vi "Digital_write_signal.vi"() -> ()   [LabVIEW 2020]
uses:
  <vilib>/DAQmx/write.llb/DAQmx Write (Digital 1D Bool NChan 1Samp 1Line).vi
  <vilib>/DAQmx/create/channels.llb/DAQmx Create Channel (DO-Digital Output).vi
  <vilib>/DAQmx/miscellaneous.llb/DAQmx Fill In Error Info.vi
panel:
  in  "Text Ring":u16(ring) items=["All Off", "488", "560", "595", "640"]
  in  "Stop":bool
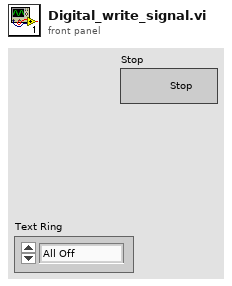
[diagram p1: front panel]
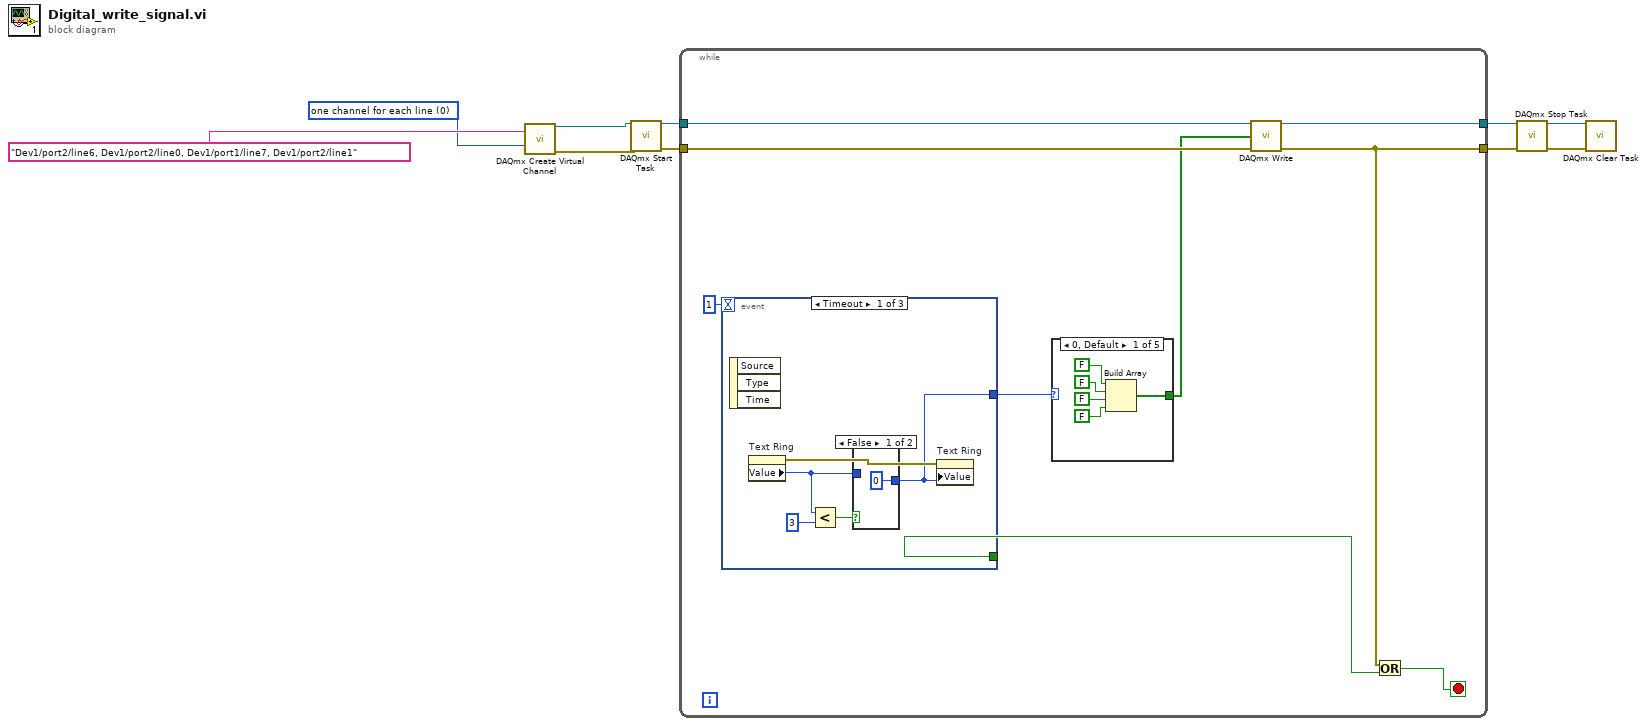
[diagram p0: block diagram]
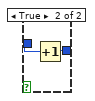
[diagram p2: hidden frame]
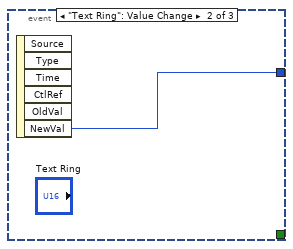
[diagram p3: hidden frame]
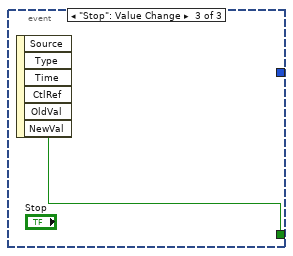
[diagram p4: hidden frame]
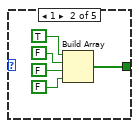
[diagram p5: hidden frame]
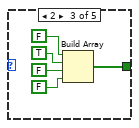
[diagram p6: hidden frame]
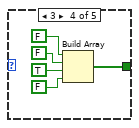
[diagram p7: hidden frame]
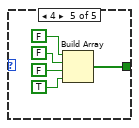
[diagram p8: hidden frame]
diagram:
  w1 = 0 items=["one channel for each line", "one channel for all lines"] ("line grouping")
  n1 = call-poly <vilib>:"DAQmx Create Virtual Channel.vi"("lines"=tag "Dev1/port2/line6, Dev1/port2/line0, Dev1/port1/line7, Dev1/port2/line1", "line grouping"=w1) -> ("task out"=w8:refnum<k21>, "error out"=w7:errorcluster)  [unwired: 12 in]
  n2 = call <vilib>:"DAQmx Start Task.vi"("task/channels in"=w8, "error in"=w7) -> ("task out"=w10:refnum<k21>, "error out"=w9:errorcluster)  [unwired: 12 in]
  n3 = while {
    tunnel: w10 -> [w19]
    tunnel: w9 -> [w18]
    tunnel: [w17] -> w6
    tunnel: [w15] -> w5
    stop <- w16 stop-if-true
    n4 = event shown="[0] Timeout" {
      selector: _ -> [_ _ _]
      dyn-events: _ -> [_ _ _]
      timeout: 1 -> [_ _ _]
      tunnel: [w20 w28 _] -> w14
      tunnel: [_ _ w29] -> w12
      event Timeout {
        n5 = event-data() -> ()  [unwired: 1 in, 3 out]
        n6 = property on="Text Ring" class="Ring (strict)"() -> (error out=w24:errorcluster, "Value"=w22:u16)  [unwired: 2 in, 1 out]
        n7 = Less?(x=w22, y=u16 3) -> (x < y?=w23:bool)
        n8 = case shown="False" w23 {
          tunnel: w22 -> [_ w27]
          tunnel: [u16 0 w26] -> w20
          frame False {
          }
          frame True {
            n9 = Increment(x=w27) -> (x+1=w26:u16)
          }
        }
        n10 = property on="Text Ring" class="Ring (strict)"(error in=w24, "Value"=w20) -> ()  [unwired: 1 in, 2 out]
      }
      event "Text Ring": Value Change {
        n11 = event-data() -> ("NewVal"=w28:u16)  [unwired: 1 in, 5 out]
      }
      event "Stop": Value Change {
        n12 = event-data() -> ("NewVal"=w29:bool)  [unwired: 1 in, 5 out]
      }
    }
    n13 = case shown="0, Default" w14 {
      tunnel: [w31 w36 w41 w46 w51] -> w13
      frame 0, Default {
        n14 = Build Array(FALSE, FALSE ("element"), FALSE ("element"), FALSE ("element")) -> (w31:bool[])
      }
      frame 1 {
        n15 = Build Array(TRUE, FALSE ("element"), FALSE ("element"), FALSE ("element")) -> (w36:bool[])
      }
      frame 2 {
        n16 = Build Array(FALSE, TRUE ("element"), FALSE ("element"), FALSE ("element")) -> (w41:bool[])
      }
      frame 3 {
        n17 = Build Array(FALSE, FALSE ("element"), TRUE ("element"), FALSE ("element")) -> (w46:bool[])
      }
      frame 4 {
        n18 = Build Array(FALSE, FALSE ("element"), FALSE ("element"), TRUE ("element")) -> (w51:bool[])
      }
    }
    n19 = call-poly <vilib>:"DAQmx Write.vi"("task/channels in"=w19, "data"=w13, "error in"=w18) -> ("task out"=w17:refnum<k21>, "error out"=w15:errorcluster)  [unwired: 10 in, 1 out]
    n20 = Or(x=w15, y=w12) -> (x .or. y?=w16:bool)
  }
  n21 = call <vilib>:"DAQmx Stop Task.vi"("task/channels in"=w6, "error in"=w5) -> ("task out"=w4:refnum<k21>, "error out"=w3:errorcluster)  [unwired: 12 in]
  n22 = call <vilib>:"DAQmx Clear Task.vi"("task in"=w4, "error in"=w3) -> ()  [unwired: 13 in, 1 out]
